vi "Seq Dialog Set or Check Numeric.vi"(8 "Segment Data":T1) -> (0 "Step Hisitory":string[](array[string]), 2 "Segment Data 2":T1)   [LabVIEW 2018]
uses:
  type defs/Sequence Info.ctl
panel:
  out "error out":errorcluster
  out "String 2":string="Pre Run Station - Glass - Vent Open"
  in  "Voltage":dbl=10.0 format="%#.2f"
  in  "Description":string
  in  "Save":bool
  in  "Cancel":bool
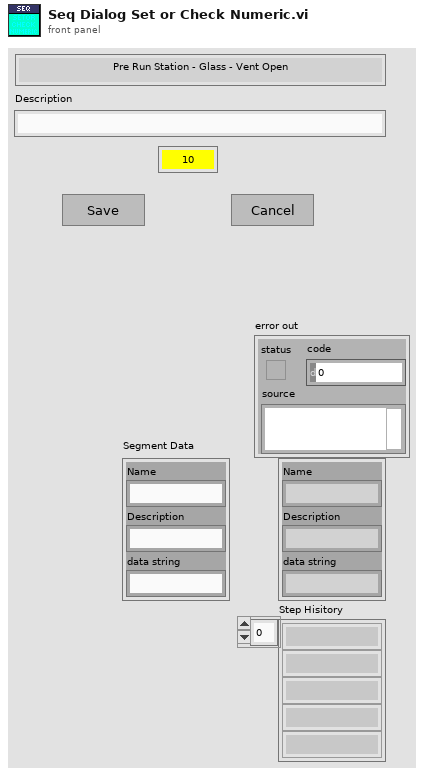
[diagram p1: front panel]
types:
  T1 = typedef "Sequence Info.ctl" = cluster{"Name":string, "Description":string, "data string":string}
  T2 = cluster{"Segment Data":T1, "Old Data":string, "New Data":string}
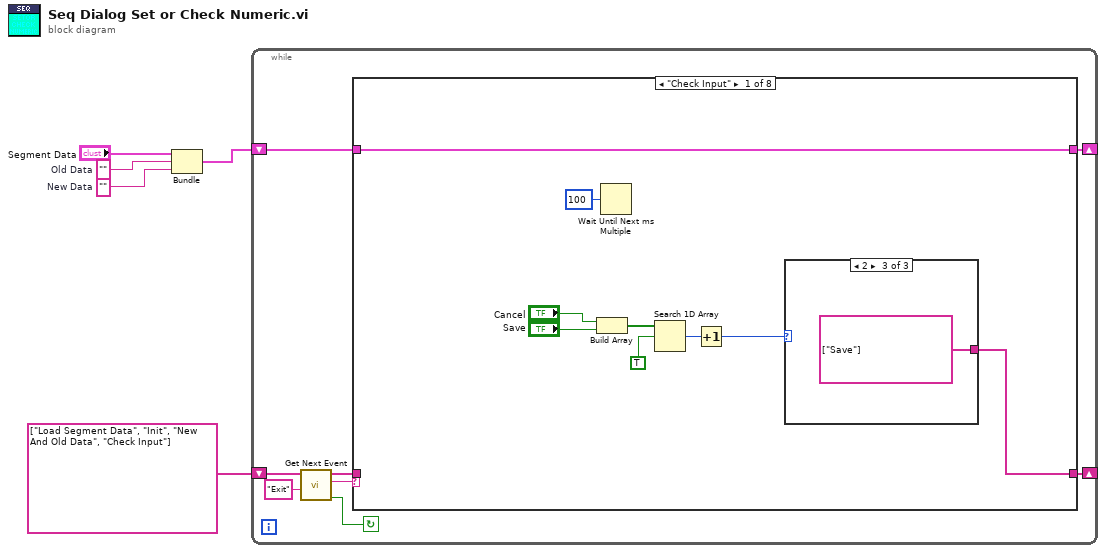
[diagram p0: block diagram]
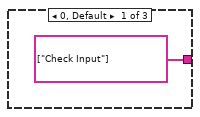
[diagram p2: hidden frame]
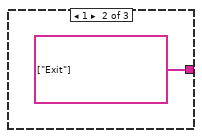
[diagram p3: hidden frame]
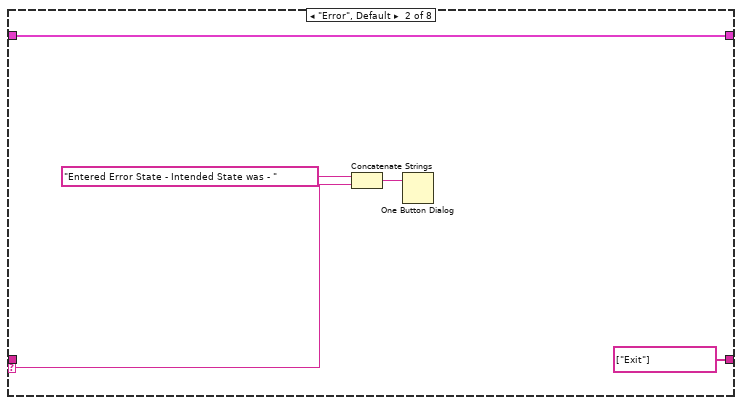
[diagram p4: hidden frame]
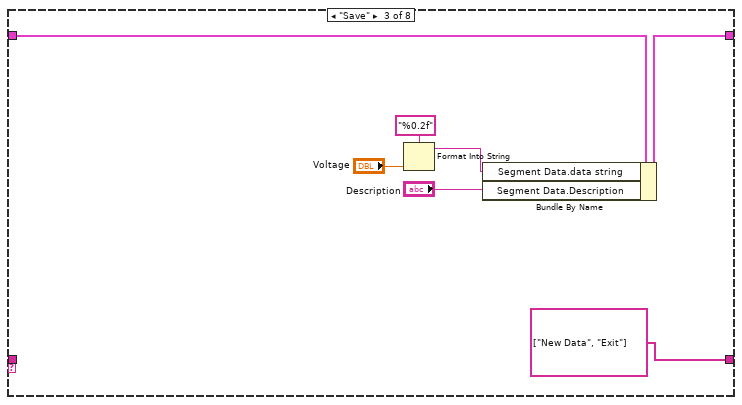
[diagram p5: hidden frame]
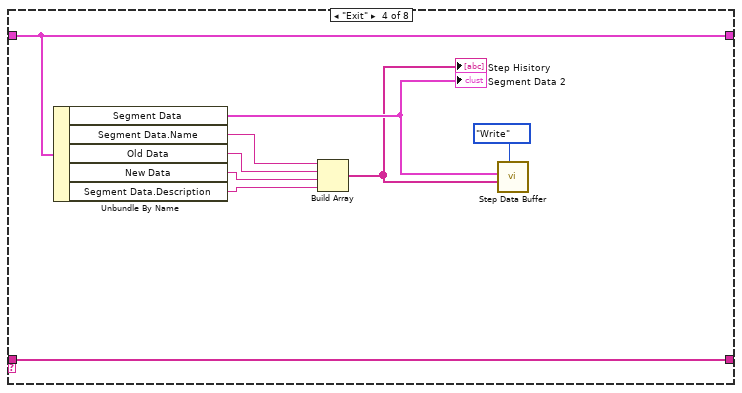
[diagram p6: hidden frame]
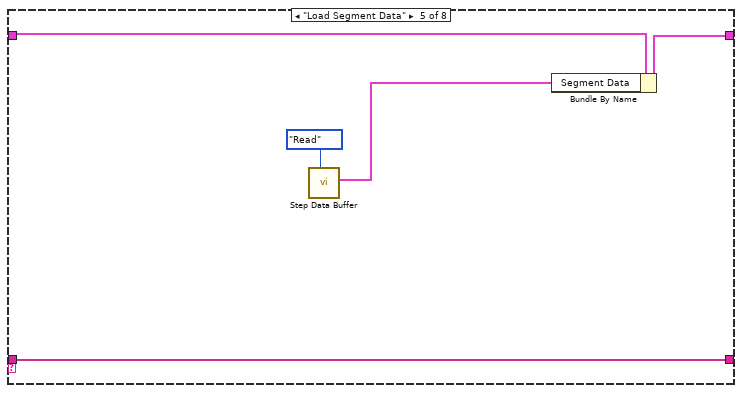
[diagram p7: hidden frame]
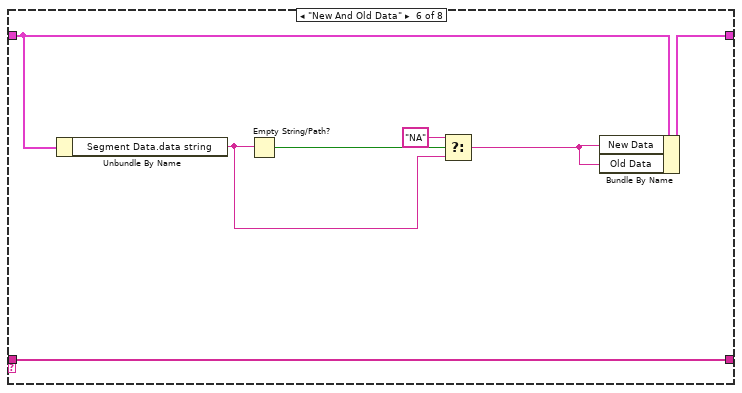
[diagram p8: hidden frame]
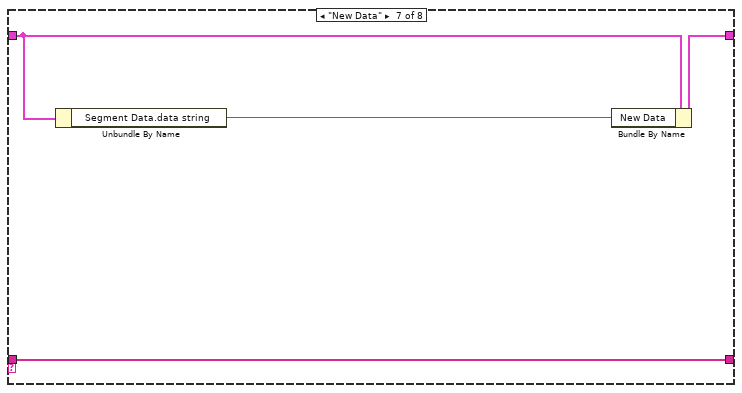
[diagram p9: hidden frame]
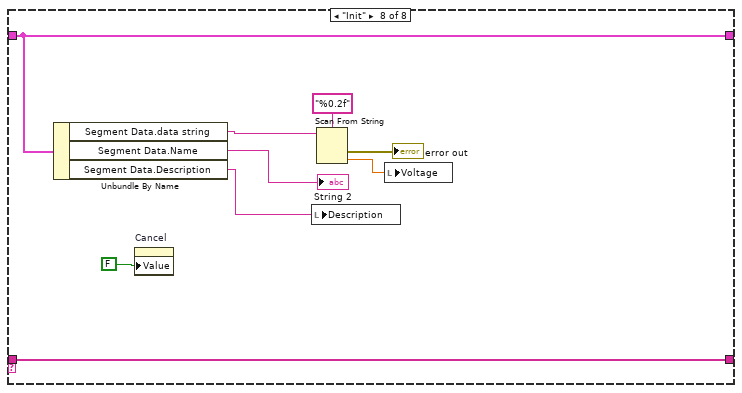
[diagram p10: hidden frame]
diagram:
  w1 = ""  # New Data
  w2 = ""  # Old Data
  n1 = Bundle("Segment Data"="Segment Data", "Old Data"=w2, "New Data"=w1) -> (w5:T2)  [unwired: 1 in]
  n2 = while {
    shift-right: [w11] -> _
    shift-left: string[] ["Load Segment Data", "Init", "New And Old Data", "Check Input"] ("Event queue out") -> [w10]
    shift-right: [w6] -> _
    shift-left: w5 -> [w7]
    stop <- w9 continue-if-true
    n3 = call "Get Next Event.vi"("Exit Event"="Exit", "event queue in"=w10) -> ("Condition (Exit:F)"=w9:bool, "next event"=w13:string, "event queue out"=w12:string[])  [unwired: 3 in]
    n4 = case shown="\"Check Input\"" w13 {
      selector: w13 -> [_ w27 _ _ _ _ _ _]
      tunnel: w12 -> [_ _ _ w46 w51 w52 w61 w71]
      tunnel: [w17 string[] ["Exit"] ("event queue out") string[] ["New Data", "Exit"] ("Event queue out") w46 w51 w52 w61 w71] -> w11
      tunnel: w7 -> [w22 w30 w33 w42 w50 w54 w59 w63]
      tunnel: [w22 w30 w37 w42 w48 w53 w60 w63] -> w6
      frame "Check Input" {
        n5 = Build Array("Cancel", "Save") -> (w19:bool[])
        n6 = Wait Until Next ms Multiple(millisecond multiple=u32 100) -> ()  [unwired: 1 out]
        n7 = Search 1D Array(1D array=w19, element=TRUE) -> (index of element=w20:i32)  [unwired: 1 in]
        n8 = Increment(x=w20) -> (x+1=w21:i32)
        n9 = case shown="2" w21 {
          tunnel: [string[] ["Check Input"] ("Events to Insert") string[] ["Exit"] ("Events to Insert") string[] ["Save"] ("Events to Insert")] -> w17
          frame 0, Default {
          }
          frame 1 {
          }
          frame 2 {
          }
        }
      }
      frame "Error", Default {
        n10 = Concatenate Strings("Entered Error State - Intended State was - " ("string"), w27) -> (w28:string)
        n11 = One Button Dialog(message=w28) -> ()  [unwired: 1 in, 1 out]
      }
      frame "Save" {
        n12 = Format Into String(format string="%0.2f", "Voltage") -> (resulting string=w34:string)  [unwired: 2 in, 1 out]
        n13 = Bundle By Name(cluster=w33, "Segment Data.data string"=w34, "Segment Data.Description"="Description") -> (w37:T2)
      }
      frame "Exit" {
        n14 = Unbundle By Name(w42) -> ("Segment Data"=w40:T1, "Segment Data.Name"=w45:string, "Old Data"=w44:string, "New Data"=w43:string, "Segment Data.Description"=w38:string)
        "Segment Data 2" <- w40
        n15 = Build Array(w45, w44, w43, w38) -> (w39:string[])
        "Step Hisitory" <- w39
        n16 = call "Step Data Buffer.vi"("Mode"=enum16{"Init", "Read", "Write"}."Write", "Step Hisitory In"=w39, "Segment Data In"=w40) -> ()  [unwired: 4 in, 5 out]
      }
      frame "Load Segment Data" {
        n17 = call "Step Data Buffer.vi"("Mode"=enum16{"Init", "Read", "Write"}."Read") -> ("Segment Data Out"=w47:T1)  [unwired: 6 in, 4 out]
        n18 = Bundle By Name(cluster=w50, "Segment Data"=w47) -> (w48:T2)
      }
      frame "New And Old Data" {
        n19 = Unbundle By Name(w54) -> ("Segment Data.data string"=w58:string)
        n20 = Empty String/Path?(string/path=w58) -> (empty?=w55:bool)
        n21 = Select(t="NA", s=w55, f=w58) -> (s? t:f=w57:string)
        n22 = Bundle By Name(cluster=w54, "New Data"=w57, "Old Data"=w57) -> (w53:T2)
      }
      frame "New Data" {
        n23 = Unbundle By Name(w59) -> ("Segment Data.data string"=w62:string)
        n24 = Bundle By Name(cluster=w59, "New Data"=w62) -> (w60:T2)
      }
      frame "Init" {
        n25 = Unbundle By Name(w63) -> ("Segment Data.data string"=w66:string, "Segment Data.Name"=→"String 2":string, "Segment Data.Description"=w65:string)
        n26 = property on="Cancel" class="Bool (严格)"("Value"=FALSE ("Cancel")) -> ()  [unwired: 2 in, 2 out]
        n27 = local write "Description"(w65) -> ()
        n28 = Scan From String(format string="%0.2f", input string=w66) -> (error out=→"error out":errorcluster, output 1=w67:dbl)  [unwired: 3 in, 2 out]
        n29 = local write "Voltage"(w67) -> ()
      }
    }
  }
